vi "Write status message.vi"(8 "error in (no error)":errorcluster, 10 "JSON message":T1, 11 "Channel in":refnum<class "SPARC4_Channel.lvclass">) -> (0 "error out":errorcluster, 3 "Channel out":refnum<class "SPARC4_Channel.lvclass">)   [LabVIEW 2018, in "SPARC4_Channel.lvclass"]
uses:
  SPARC4_Channel.lvclass
  SPARC4_Channel.lvclass/SPARC4_Channel.ctl
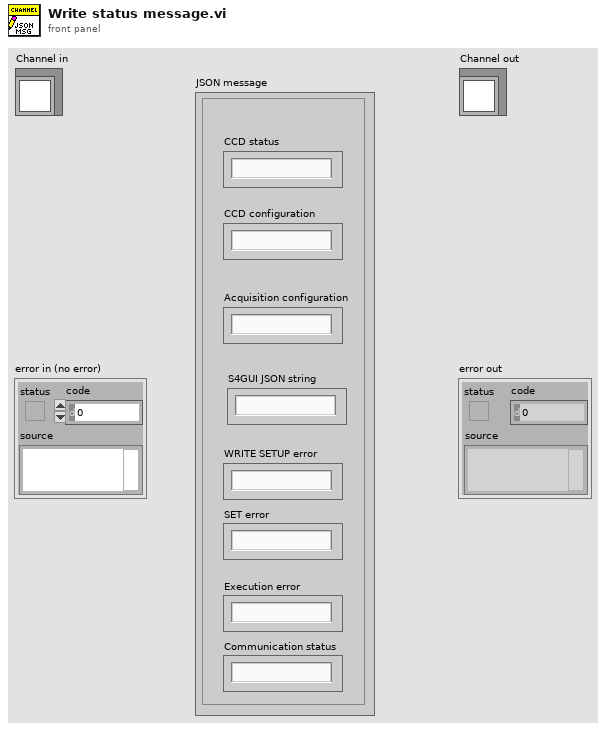
[diagram p1: front panel]
types:
  T1 = cluster{"CCD status":string, "CCD configuration":string, "Acquisition configuration":string, "S4GUI JSON string":string, "WRITE SETUP error":string, "Execution error":string, "SET error":string, "Communication status":string}
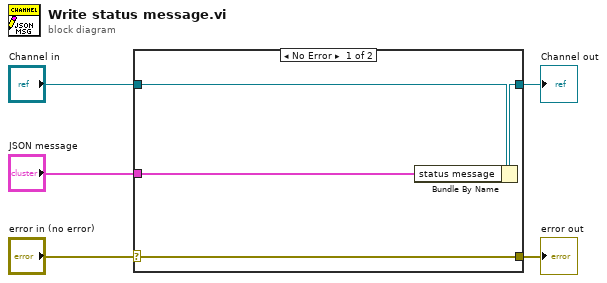
[diagram p0: block diagram]
diagram:
  n1 = case shown="No Error" "error in (no error)" {
    selector: "error in (no error)" -> [w9 w10]
    tunnel: [w9 w10] -> w4
    tunnel: [w7 w11] -> w2
    tunnel: "Channel in" -> [w8 w11]
    tunnel: "JSON message" -> [w6 _]
    frame No Error {
      n2 = Bundle By Name(cluster=w8, "status message"=w6) -> (w7:refnum<class "SPARC4_Channel.lvclass">)
    }
    frame Error {
    }
  }
  "error out" <- w4
  "Channel out" <- w2
